vi "IsModeAllowed.vi"(8 "error in (no error)":errorcluster, 10 "Mode":u16, 11 "PS Control Actor in":refnum<class "PS Control Actor.lvclass">) -> (0 "error out":errorcluster, 2 "Allowed":bool, 3 "PS Control Actor out":refnum<class "PS Control Actor.lvclass">)   [LabVIEW 2020, in "PS Control Actor.lvlib" / "PS Control Actor.lvclass"]
uses:
  PS Control Actor.lvclass
  PS Control Actor.lvclass/PS Control Actor.ctl
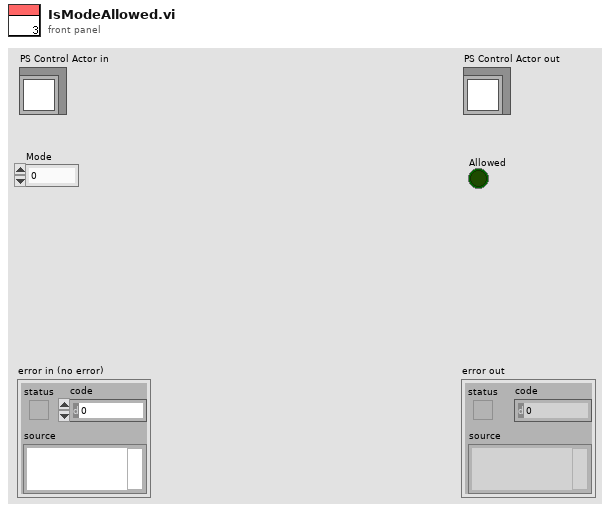
[diagram p1: front panel]
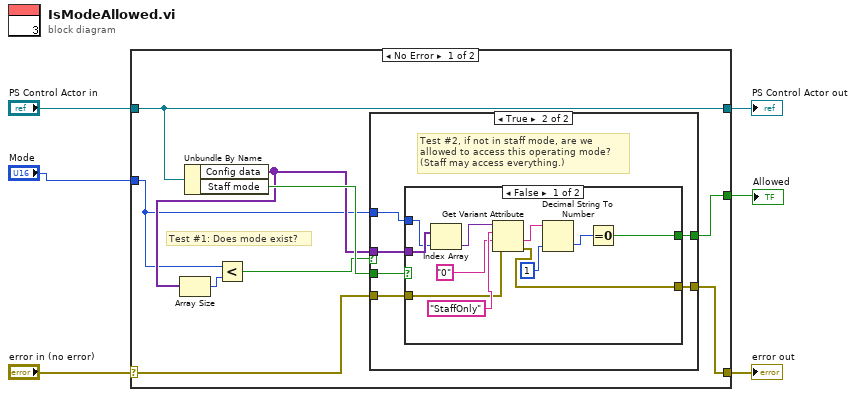
[diagram p0: block diagram]
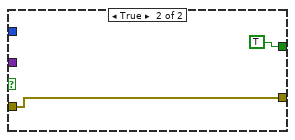
[diagram p3: hidden frame]
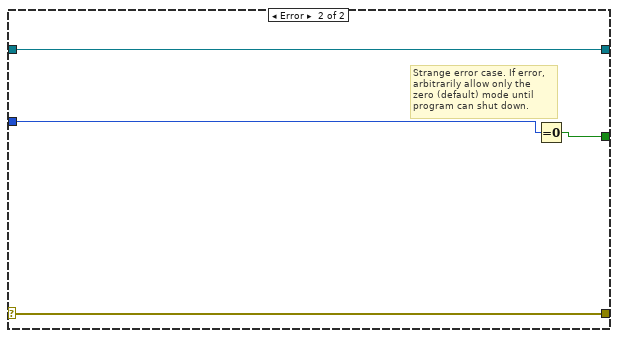
[diagram p4: hidden frame]
diagram:
  n1 = case shown="No Error" "error in (no error)" {
    selector: "error in (no error)" -> [w15 w40]
    tunnel: [w14 w40] -> w5
    tunnel: [w12 w39] -> w3
    tunnel: "PS Control Actor in" -> [w12 w39]
    tunnel: "Mode" -> [w7 w37]
    tunnel: [w11 w38] -> w1
    frame No Error {
      # "Test #1: Does mode exist?"
      n2 = Unbundle By Name(w12) -> ("Config data"=w9:variant[], "Staff mode"=w13:bool)
      n3 = Array Size(array=w9) -> (size(s)=w10:i32)
      n4 = Less?(x=w7, y=w10) -> (x < y?=w8:bool)
      n5 = case shown="True" w8 {
        selector: w8 -> [w17 _]
        tunnel: w15 -> [w16 w23]
        tunnel: [w16 w22] -> w14
        tunnel: w13 -> [_ w21]
        tunnel: [w17 w20] -> w11
        tunnel: w9 -> [_ w19]
        tunnel: w7 -> [_ w18]
        frame False {
        }
        frame True {
          # "Test #2, if not in staff mode, are we\nallowed to access this operating mode?\n(Staff may access everything.)"
          n6 = case shown="False" w21 {
            tunnel: w18 -> [w26 _]
            tunnel: w19 -> [w34 _]
            tunnel: w23 -> [w30 w36]
            tunnel: [w25 w36] -> w22
            tunnel: [w24 TRUE] -> w20
            frame False {
              n7 = Index Array(array=w34, index=w26) -> (element=w33:variant)
              n8 = Get Variant Attribute(Variant=w33, name="StaffOnly", default value (empty Variant)="0", error in=w30) -> (value=w29:string, error out=w25:errorcluster)  [unwired: 2 out]
              n9 = Decimal String To Number(string=w29, default (0L)=1 ("default (0 I32)")) -> (number=w27:i32)  [unwired: 1 in, 1 out]
              n10 = Equal To 0?(x=w27) -> (x = 0?=w24:bool)
            }
            frame True {
            }
          }
        }
      }
    }
    frame Error {
      # "Strange error case. If error,\narbitrarily allow only the\nzero (default) mode until\nprogram can shut down."
      n11 = Equal To 0?(x=w37) -> (x = 0?=w38:bool)
    }
  }
  "error out" <- w5
  "PS Control Actor out" <- w3
  "Allowed" <- w1
